vi "set_open_closed_pixels.vi"(7 "number of offset pixels":i32, 8 "error in (no error)":errorcluster, 9 "number of closed pixels":i32, 10 "number of open pixels":i32, 11 "TrajectoryDL090201FrameScan in":refnum<class "TrajectoryDL090201FrameScan.lvclass">) -> (0 "error out":errorcluster, 3 "TrajectoryDL090201FrameScan out":refnum<class "TrajectoryDL090201FrameScan.lvclass">)   [LabVIEW 2010, in "TrajectoryDL090201FrameScan.lvclass"]
uses:
  TrajectoryDL090201FrameScan.lvclass
  TrajectoryDL090201FrameScan.lvclass/TrajectoryDL090201FrameScan.ctl
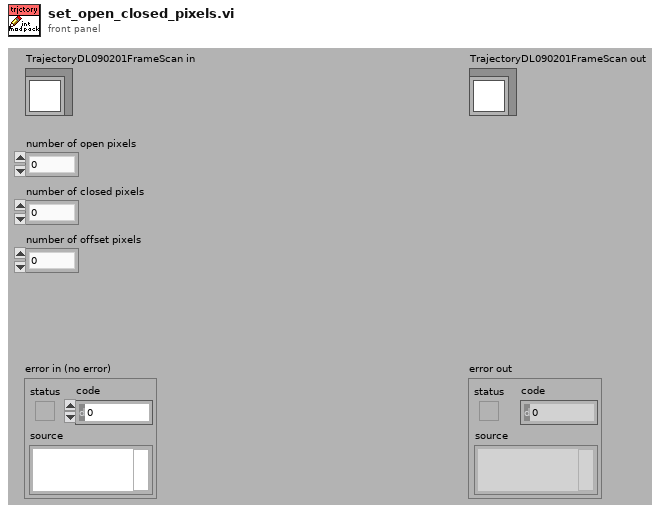
[diagram p1: front panel]
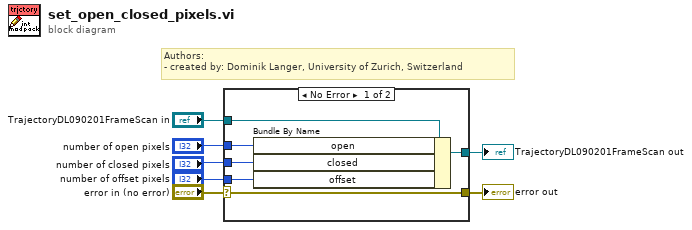
[diagram p0: block diagram]
diagram:
  # "Authors: \n- created by: Dominik Langer, University of Zurich, Switzerland"
  n1 = case shown="No Error" "error in (no error)" {
    selector: "error in (no error)" -> [w13 w15]
    tunnel: [w13 w15] -> w6
    tunnel: [w11 w14] -> w4
    tunnel: "TrajectoryDL090201FrameScan in" -> [w12 w14]
    tunnel: "number of open pixels" -> [w10 _]
    tunnel: "number of closed pixels" -> [w9 _]
    tunnel: "number of offset pixels" -> [w8 _]
    frame No Error {
      n2 = Bundle By Name(cluster=w12, "open"=w10, "closed"=w9, "offset"=w8) -> (w11:refnum<class "TrajectoryDL090201FrameScan.lvclass">)
    }
    frame Error {
    }
  }
  "error out" <- w6
  "TrajectoryDL090201FrameScan out" <- w4
